vi "Get New Mentions - Finite.vi"() -> ()   [LabVIEW 2011]
doc: "This example gets a finite number of new mentions starting from the top of the user's timeline. This example behaves the same way as Get Old Mentions- Finte if the Twitter Handle is not saved to a shift register.s"
uses:
  Controls/Tweet.ctl
  i3-twitter.lvlib
panel:
  out "Mentions Read":T1[](array[typedef])
  out "Time Stamp of Newest Mention":timestamp
  out "Num of Mentions Read":i32
  in  "Num of Mentions to Read":i32
  in  "Consumer Key":string
  in  "Consumer Secret":string
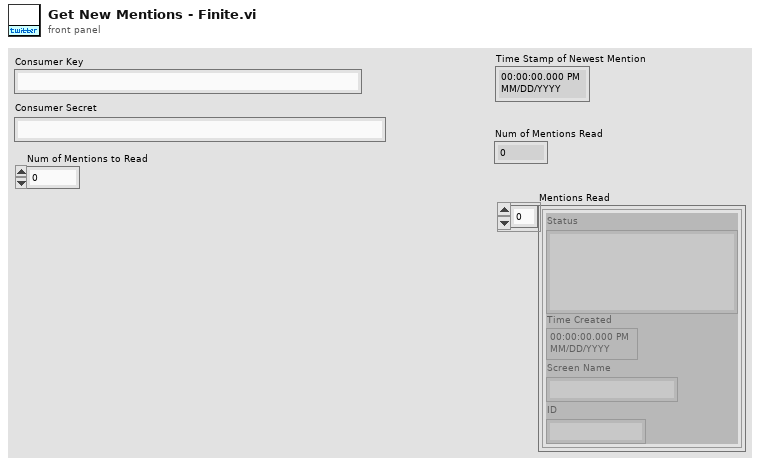
[diagram p1: front panel]
types:
  T1 = typedef "i3-twitter.lvlib/Tweet.ctl" = cluster{"Status":string, "Time Created":timestamp, "Screen Name":string, "ID":string}
  T2 = typedef "i3-twitter.lvlib/Twitter Handle.ctl" = cluster{"OAuth Credentials":T3, "since ID":string, "max ID":string, "Screen Name":string}
  T3 = typedef "i3-oauth.lvlib/OAuth Handle.ctl" = cluster{"Signature Method":T4, "Version":string, "Client":T5, "Access":T5}
  T4 = typedef "i3-oauth.lvlib/Signature Method.ctl" = enum16{"HMAC-MD5", "HMAC-SHA1", "HMAC-SHA224", "HMAC-SHA256", "HMAC-SHA384", "HMAC-SHA512"}
  T5 = typedef "i3-oauth.lvlib/Credentials.ctl" = cluster{"Token":string, "Secret":string}
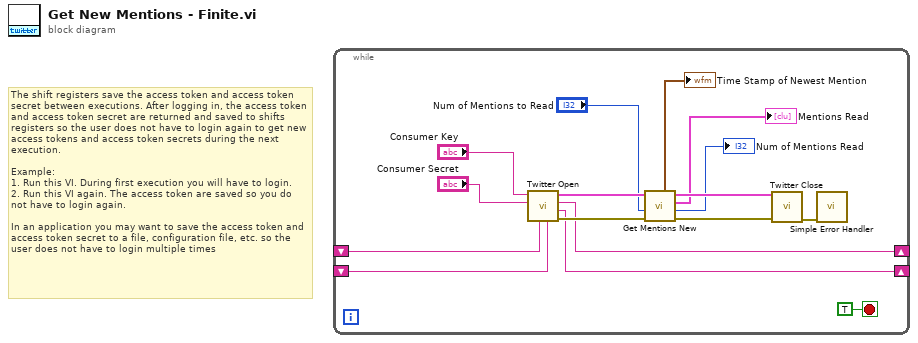
[diagram p0: block diagram]
diagram:
  # "The shift registers save the access token and access token secret between executions. After logging in, the access token and access token secret are returned and saved to shifts registers so the user does not have to login again to get new access tokens and access token secrets during the next execution.\n\nExample:\n1. Run this VI. During first execution you will have to login.\n2. Run this VI again. The access token are saved so you do not have to login again.\n\nIn an application you may want to save the access token and access token secret to a file, configuration file, etc. so the user does not have to login multiple times"
  n1 = while {
    shift-right: [w3] -> _
    shift-left: _ -> [w5]
    shift-right: [w2] -> _
    shift-left: _ -> [w4]
    stop <- TRUE stop-if-true
    n2 = call "Twitter Open.vi"("Access Token Secret (In)"=w4, "Access Token (In)"=w5, "Consumer Secret"="Consumer Secret", "Consumer Key"="Consumer Key") -> ("error out"=w11:errorcluster, "Access Token Secret (Out)"=w2:string, "Access Token (Out)"=w3:string, "Twitter Handle Out"=w14:T2)  [unwired: 4 in]
    n3 = call "Get Mentions New.vi"("error in"=w11, "Mentions to Read (10)"="Num of Mentions to Read", "Twitter Handle In"=w14) -> ("error out"=w13:errorcluster, "Actual Num of Mentions Read"=→"Num of Mentions Read":i32, "New Mentions Read"=→"Mentions Read":T1[], "Twitter Handle Out"=w12:T2, "Time Stamp of Newest Mention"=→"Time Stamp of Newest Mention":timestamp)  [unwired: 4 in]
    n4 = call "Twitter Close.vi"("error in"=w13, "Twitter Handle In"=w12) -> ("error in"=w7:errorcluster)  [unwired: 9 in]
    n5 = call <vilib>:"Simple Error Handler.vi"("error in (no error)"=w7) -> ()  [unwired: 4 in, 5 out]
  }
